vi "LVFinal-backup1.vi"() -> ()   [LabVIEW 2016]
panel:
  out "Ball Color":string[](array[string])
  out "Ball Y":dbl[](array[numeric])
  out "Ball X":dbl[](array[numeric])
  in  "Send Button":bool
  in  "DAC2":dbl
  in  "DAC1":dbl
  out "Angle":dbl
  out "Velocity":dbl
  out "Y":dbl
  out "X":dbl
  in  "stop":bool
  in  "Display History":bool
  out "2D Picture":picture
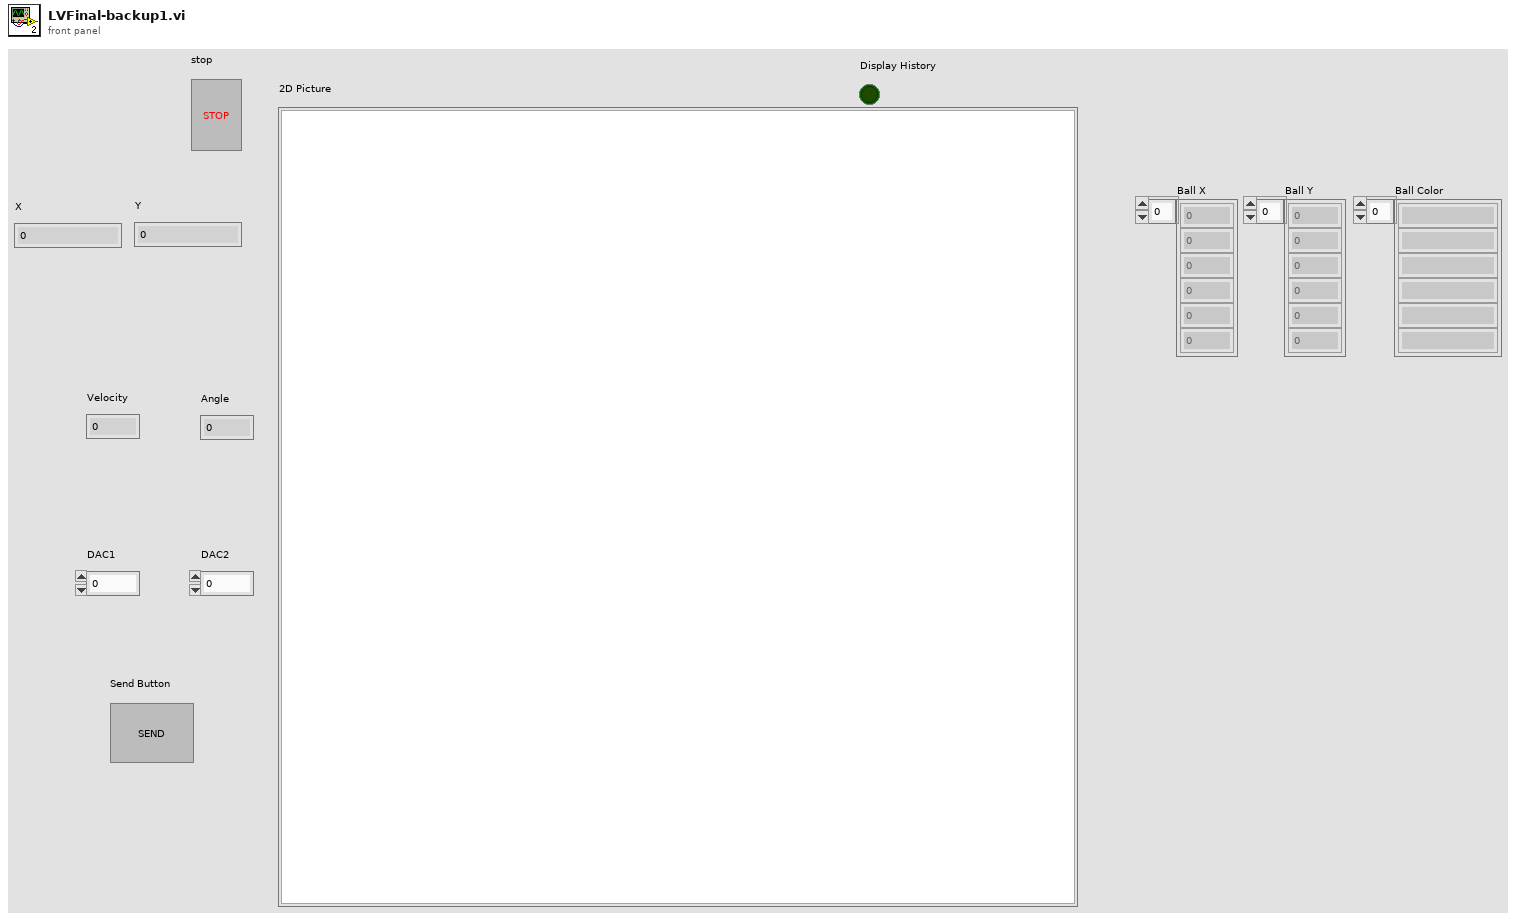
[diagram p1: front panel]
types:
  T1 = cluster{"Width":u16, "Style":enum32{"Solid", "Dash", "Dot", "DashDot", "DashDotDot"}}
  T2 = enum16{"Standard", "Buffered", "CRLF", "Immediate"}
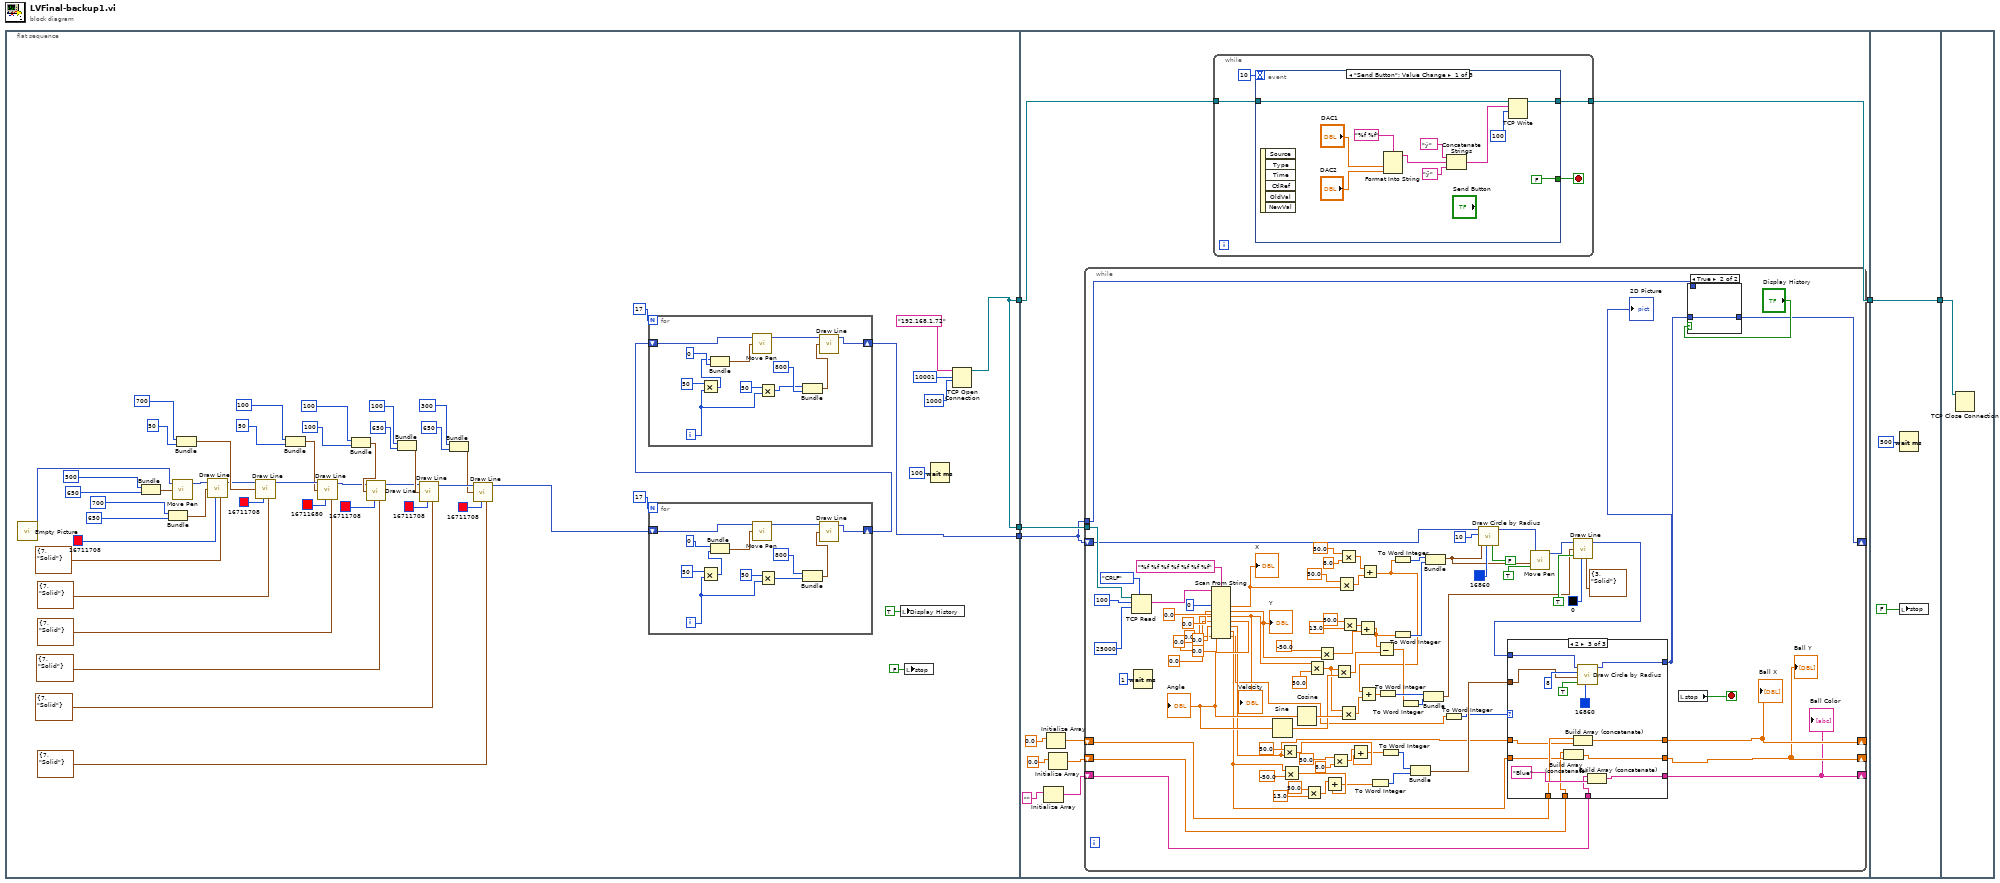
[diagram p0: block diagram]
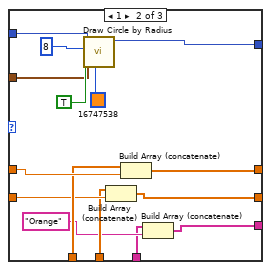
[diagram p3: hidden frame]
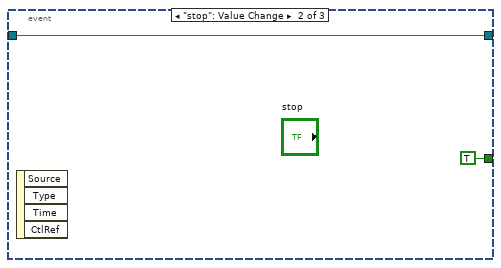
[diagram p5: hidden frame]
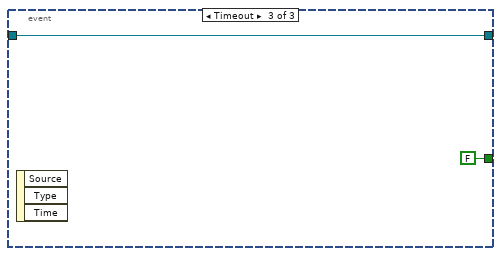
[diagram p6: hidden frame]
diagram:
  n1 = flat-sequence {
    tunnel: [w51] -> w5
    tunnel: [w47] -> w2
    tunnel: [w51] -> w1
    tunnel: w5 -> [w91]
    tunnel: [w90] -> w3
    tunnel: w2 -> [w88]
    tunnel: w1 -> [w89]
    tunnel: [w233] -> w4
    tunnel: w3 -> [w233]
    tunnel: w4 -> [w236]
    frame #0 {
      n2 = call "Empty Picture"() -> ("empty picture"=w39:picture)
      n3 = Bundle(500, 650) -> (w46:cluster{i32, i32})  [unwired: 1 in]
      n4 = Bundle(700, 650) -> (w40:cluster{i32, i32})  [unwired: 1 in]
      n5 = call <vilib>:"Move Pen.vi"("new position"=w46, "picture"=w39) -> ("new picture"=w43:picture)  [unwired: 3 in]
      n6 = Bundle(700, 50) -> (w36:cluster{i32, i32})  [unwired: 1 in]
      n7 = call <vilib>:"Draw Line.vi"("picture"=w43, "end point"=w40, "color(black)"=u32 16711708, "pen"=T1 {"Width"=7, "Style"=enum."Solid"}) -> ("new picture"=w31:picture)  [unwired: 5 in]
      n8 = call <vilib>:"Draw Line.vi"("picture"=w31, "end point"=w36, "color(black)"=u32 16711708, "pen"=T1 {"Width"=7, "Style"=enum."Solid"}) -> ("new picture"=w30:picture)  [unwired: 5 in]
      n9 = Bundle(100, 50) -> (w27:cluster{i32, i32})  [unwired: 1 in]
      n10 = call <vilib>:"Draw Line.vi"("picture"=w30, "end point"=w27, "color(black)"=u32 16711680, "pen"=T1 {"Width"=7, "Style"=enum."Solid"}) -> ("new picture"=w21:picture)  [unwired: 5 in]
      n11 = Bundle(100, 100) -> (w22:cluster{i32, i32})  [unwired: 1 in]
      n12 = call <vilib>:"Draw Line.vi"("picture"=w21, "end point"=w22, "color(black)"=u32 16711708, "pen"=T1 {"Width"=7, "Style"=enum."Solid"}) -> ("new picture"=w17:picture)  [unwired: 5 in]
      n13 = Bundle(100, 650) -> (w18:cluster{i32, i32})  [unwired: 1 in]
      n14 = call <vilib>:"Draw Line.vi"("picture"=w17, "end point"=w18, "color(black)"=u32 16711708, "pen"=T1 {"Width"=7, "Style"=enum."Solid"}) -> ("new picture"=w12:picture)  [unwired: 5 in]
      n15 = Bundle(300, 650) -> (w11:cluster{i32, i32})  [unwired: 1 in]
      n16 = call <vilib>:"Draw Line.vi"("picture"=w12, "end point"=w11, "color(black)"=u32 16711708, "pen"=T1 {"Width"=7, "Style"=enum."Solid"}) -> ("new picture"=w6:picture)  [unwired: 5 in]
      n17 = for {
        N: 17 -> [_]
        shift-right: [w70] -> w48
        shift-left: w6 -> [w72]
        i -> [w71]
        n18 = Multiply(x=50, y=w71) -> (x*y=w74:i32)
        n19 = Bundle(0, w74) -> (w73:cluster{i32, i32})  [unwired: 1 in]
        n20 = call <vilib>:"Move Pen.vi"("new position"=w73, "picture"=w72) -> ("new picture"=w81:picture)  [unwired: 3 in]
        n21 = Multiply(x=50, y=w71) -> (x*y=w79:i32)
        n22 = Bundle(800, w79) -> (w77:cluster{i32, i32})  [unwired: 1 in]
        n23 = call <vilib>:"Draw Line.vi"("picture"=w81, "end point"=w77) -> ("new picture"=w70:picture)  [unwired: 7 in]
      }
      n24 = for {
        N: 17 -> [_]
        shift-right: [w62] -> w47
        shift-left: w48 -> [w64]
        i -> [w63]
        n25 = Multiply(x=50, y=w63) -> (x*y=w60:i32)
        n26 = Bundle(w60, 0) -> (w65:cluster{i32, i32})  [unwired: 1 in]
        n27 = call <vilib>:"Move Pen.vi"("new position"=w65, "picture"=w64) -> ("new picture"=w69:picture)  [unwired: 3 in]
        n28 = Multiply(x=50, y=w63) -> (x*y=w58:i32)
        n29 = Bundle(w58, 800) -> (w67:cluster{i32, i32})  [unwired: 1 in]
        n30 = call <vilib>:"Draw Line.vi"("picture"=w69, "end point"=w67) -> ("new picture"=w62:picture)  [unwired: 7 in]
      }
      n31 = local write "Display History"(TRUE ("Display History")) -> ()
      n32 = local write "stop"(FALSE ("stop")) -> ()
      n33 = Wait (ms)(milliseconds to wait=u32 100) -> ()  [unwired: 1 out]
      n34 = TCP Open Connection(address="192.168.1.72", remote port or service name=u16 10001, timeout ms (60000)=1000) -> (connection ID=w51:refnum<k5>)  [unwired: 2 in, 1 out]
    }
    frame #1 {
      n35 = Initialize Array("") -> (w83:string[])  [unwired: 1 in]
      n36 = Initialize Array(0.0 ("element")) -> (w87:dbl[])  [unwired: 1 in]
      n37 = Initialize Array(0.0 ("element")) -> (w84:dbl[])  [unwired: 1 in]
      n38 = while {
        shift-right: [w164] -> _
        shift-left: w88 -> [w152]
        tunnel: w89 -> [w163]
        tunnel: w88 -> [w162]
        shift-right: [w99] -> _
        shift-left: w84 -> [w100]
        shift-right: [w101] -> _
        shift-left: w87 -> [w102]
        shift-right: [w97] -> _
        shift-left: w83 -> [w98]
        stop <- w177 stop-if-true
        n39 = TCP Read(connection ID=w163, bytes to read=100, 7:T2."CRLF" ("mode (standard)"), 9:25000 ("timeout ms (25000)")) -> (data out=w172:string)  [unwired: 1 in, 2 out]
        n40 = Wait (ms)(milliseconds to wait=u32 1) -> ()  [unwired: 1 out]
        n41 = Scan From String(format string="%f %f %f %f %f %f %f", input string=w172, initial scan location=u32 0, default 1=0.0 ("default value 1"), default 2=0.0 ("default value 2"), default 3=0.0 ("default value 3"), default 4=0.0 ("default value 4"), default 5=0.0 ("default value 5"), default 6=0.0 ("default value 6"), default 7=0.0 ("default value 7")) -> (output 1=w137:dbl, output 2=w132:dbl, output 3=w92:dbl, output 4=w145:dbl, output 5=w96:dbl, output 6=w95:dbl, output 7=w93:dbl)  [unwired: 1 in, 3 out]
        "X" <- w137
        "Y" <- w132
        "Velocity" <- w92
        "Angle" <- w145
        n42 = Sine(x=w145) -> (sin(x)=w144:dbl)
        n43 = Multiply(x=50.0, y=w96) -> (x*y=w112:dbl)
        n44 = Multiply(x=w95, y=-50.0) -> (x*y=w116:dbl)
        n45 = Cosine(x=w145) -> (cos(x)=w146:dbl)
        n46 = Multiply(x=50.0, y=13.0) -> (x*y=w117:dbl)
        n47 = Multiply(x=w92, y=50.0 ("x")) -> (x*y=w125:dbl)
        n48 = Multiply(x=-50.0, y=w132) -> (x*y=w127:dbl)
        n49 = Add(x=w117, y=w116) -> (x+y=w104:dbl)
        n50 = Multiply(x=50.0, y=8.0) -> (x*y=w113:dbl)
        n51 = Multiply(x=w125, y=w144) -> (x*y=w141:dbl)
        n52 = Multiply(x=50.0, y=w137) -> (x*y=w136:dbl)
        n53 = Multiply(x=50.0, y=8.0) -> (x*y=w133:dbl)
        n54 = Multiply(x=w125, y=w146) -> (x*y=w143:dbl)
        n55 = Multiply(x=50.0, y=13.0) -> (x*y=w129:dbl)
        n56 = Add(x=w113, y=w112) -> (x+y=w103:dbl)
        n57 = Add(x=w129, y=w127) -> (x+y=w126:dbl)
        n58 = Add(x=w133, y=w136) -> (x+y=w128:dbl)
        n59 = Add(x=w128, y=w143) -> (x+y=w142:dbl)
        n60 = To Word Integer(number=w104) -> (16bit integer=w110:i16)
        n61 = Subtract(x=w126, y=w141) -> (x-y=w140:dbl)
        n62 = To Word Integer(number=w142) -> (16bit integer=w154:i16)
        n63 = To Word Integer(number=w103) -> (16bit integer=w111:i16)
        n64 = To Word Integer(number=w126) -> (16bit integer=w148:i16)
        n65 = To Word Integer(number=w128) -> (16bit integer=w161:i16)
        n66 = To Word Integer(number=w140) -> (16bit integer=w147:i16)
        n67 = Bundle(w111, w110) -> (w109:cluster{i16, i16})  [unwired: 1 in]
        n68 = Bundle(w154, w147) -> (w149:cluster{i16, i16})  [unwired: 1 in]
        n69 = Bundle(w161, w148) -> (w122:cluster{i16, i16})  [unwired: 1 in]
        n70 = To Word Integer(number=w93) -> (16bit integer=w106:i16)
        n71 = call <vilib>:"Draw Circle by Radius.vi"("color(black)"=u32 16860, "fill?(F)"=FALSE, "pixel center"=w122, "radius"=i16 10, "picture"=w152) -> ("new picture"=w151:picture)  [unwired: 6 in]
        n72 = call <vilib>:"Move Pen.vi"("absolute coordinates?(T)"=TRUE, "new position"=w122, "picture"=w151) -> ("new picture"=w150:picture)  [unwired: 2 in]
        n73 = call <vilib>:"Draw Line.vi"("picture"=w150, "end point"=w149, "absolute coordinates?(T)"=TRUE, "color(black)"=u32 0, "pen"=T1 {"Width"=3, "Style"=enum."Solid"}) -> ("new picture"=w124:picture)  [unwired: 4 in]
        n74 = case shown="2" w106 {
          tunnel: w124 -> [w181 w196 w208]
          tunnel: [w181 w195 w207] -> w123
          tunnel: w109 -> [_ w192 w206]
          tunnel: w95 -> [_ w187 w199]
          tunnel: [w180 w185 w203] -> w99
          tunnel: [w179 w188 w202] -> w101
          tunnel: w96 -> [_ w190 w200]
          tunnel: [w178 w182 w204] -> w97
          tunnel: w102 -> [w179 w189 w201]
          tunnel: w100 -> [w180 w186 w198]
          tunnel: w98 -> [w178 w183 w197]
          frame 0, Default {
          }
          frame 1 {
            n75 = call <vilib>:"Draw Circle by Radius.vi"("color(black)"=u32 16747538, "fill?(F)"=TRUE, "pixel center"=w192, "radius"=i16 8, "picture"=w196) -> ("new picture"=w195:picture)  [unwired: 6 in]
            n76 = Build Array (concatenate)(w186, w187) -> (w185:dbl[])
            n77 = Build Array (concatenate)(w189, w190) -> (w188:dbl[])
            n78 = Build Array (concatenate)(w183, "Orange") -> (w182:string[])
          }
          frame 2 {
            n79 = Build Array (concatenate)(w198, w199) -> (w203:dbl[])
            n80 = Build Array (concatenate)(w201, w200) -> (w202:dbl[])
            n81 = call <vilib>:"Draw Circle by Radius.vi"("color(black)"=u32 16860, "fill?(F)"=TRUE, "pixel center"=w206, "radius"=i16 8, "picture"=w208) -> ("new picture"=w207:picture)  [unwired: 6 in]
            n82 = Build Array (concatenate)(w197, "Blue") -> (w204:string[])
          }
        }
        "2D Picture" <- w123
        "Ball X" <- w101
        "Ball Y" <- w99
        "Ball Color" <- w97
        n83 = local read "stop"() -> (w177:bool)
        n84 = case shown="True" "Display History" {
          tunnel: w123 -> [_ w213]
          tunnel: [w212 w213] -> w164
          tunnel: w162 -> [w212 _]
          frame False {
          }
          frame True {
          }
        }
      }
      n85 = while {
        tunnel: w91 -> [w216]
        tunnel: [w215] -> w90
        stop <- w217 stop-if-true
        n86 = event shown="[0] \"Send Button\": Value Change" {
          selector: _ -> [_ _ _]
          dyn-events: _ -> [_ _ _]
          timeout: 10 -> [_ _ _]
          tunnel: [FALSE TRUE FALSE] -> w217
          tunnel: w216 -> [w219 w229 w232]
          tunnel: [w218 w229 w232] -> w215
          event "Send Button": Value Change {
            n87 = event-data() -> ()  [unwired: 1 in, 6 out]
            n88 = Format Into String(format string="%f %f", "DAC1", "DAC2") -> (resulting string=w226:string)  [unwired: 2 in, 1 out]
            n89 = Concatenate Strings("ý" ("string"), w226, "ÿ" ("string")) -> (w221:string)
            n90 = TCP Write(connection ID=w219, data in=w221, 9:100 ("timeout ms (25000)")) -> (connection ID out=w218:refnum<k5>)  [unwired: 1 in, 2 out]
          }
          event "stop": Value Change {
            n91 = event-data() -> ()  [unwired: 1 in, 4 out]
          }
          event Timeout {
            n92 = event-data() -> ()  [unwired: 1 in, 3 out]
          }
        }
      }
    }
    frame #2 {
      n93 = Wait (ms)(milliseconds to wait=u32 500) -> ()  [unwired: 1 out]
      n94 = local write "stop"(FALSE) -> ()
    }
    frame #3 {
      n95 = TCP Close Connection(connection ID=w236) -> ()  [unwired: 2 in, 2 out]
    }
  }
